vi "Show Front Panel.vi"(4 "Window Vertical Size (pixels)":i16=600, 6 "Window Horizontal Size (pixels)":i16=800, 8 "Error In":errorcluster, 10 "Window Behaviour":T1, 11 "VI Reference":refnum<vi>) -> (0 "Error Out":errorcluster)   [LabVIEW 2016, in "Error Manager.lvlib"]
doc: "This VI configures the front panel window of the Error Manager Main VI. This VI is expected to be called when the user presses the button that enables them to view the list of errors that may have occurred in the application up to that point."
uses:
  Error Manager.lvlib
  <vilib>/Utility/miscctls.llb/LVPointTypeDef.ctl
  <vilib>/Utility/miscctls.llb/LVRectTypeDef.ctl
  Settings/Window_Behaviour (enum).ctl
  Settings/Settings.lvclass
panel:
  # "Development\ncontrols/indicators useful for development and testing, but which are not outputs of the VI"
  # "Input\nInputs to the VI"
  # "Output\nOutputs of the VI"
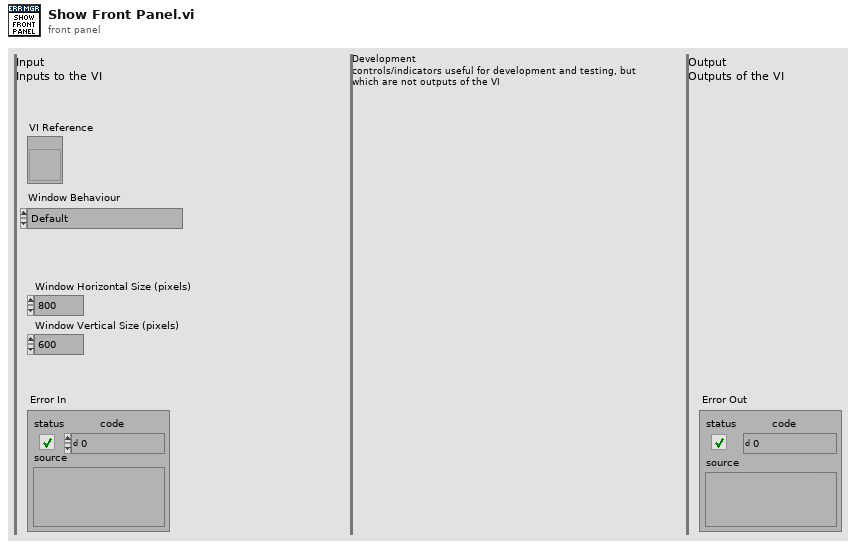
[diagram p1: front panel]
types:
  T1 = typedef "Error Manager.lvlib/Settings.lvclass/Window_Behaviour (enum).ctl" = enum16{"Default", "Floating", "Modal"}
  T2 = enum32{"Invalid", "Standard", "Closed", "Hidden", "Minimized", "Maximized"}
  T3 = typedef "LVRectTypeDef.ctl" = cluster{"Left":i16, "Top":i16, "Right":i16, "Bottom":i16}
  T4 = typedef "LVPointTypeDef.ctl" = cluster{"Horizontal":i16, "Vertical":i16}
  T5 = enum16{"Always On", "Always Off", "Off While Running"}
  T6 = enum32{"Invalid", "Default", "Floating", "Floating/Auto-Hide", "Modal"}
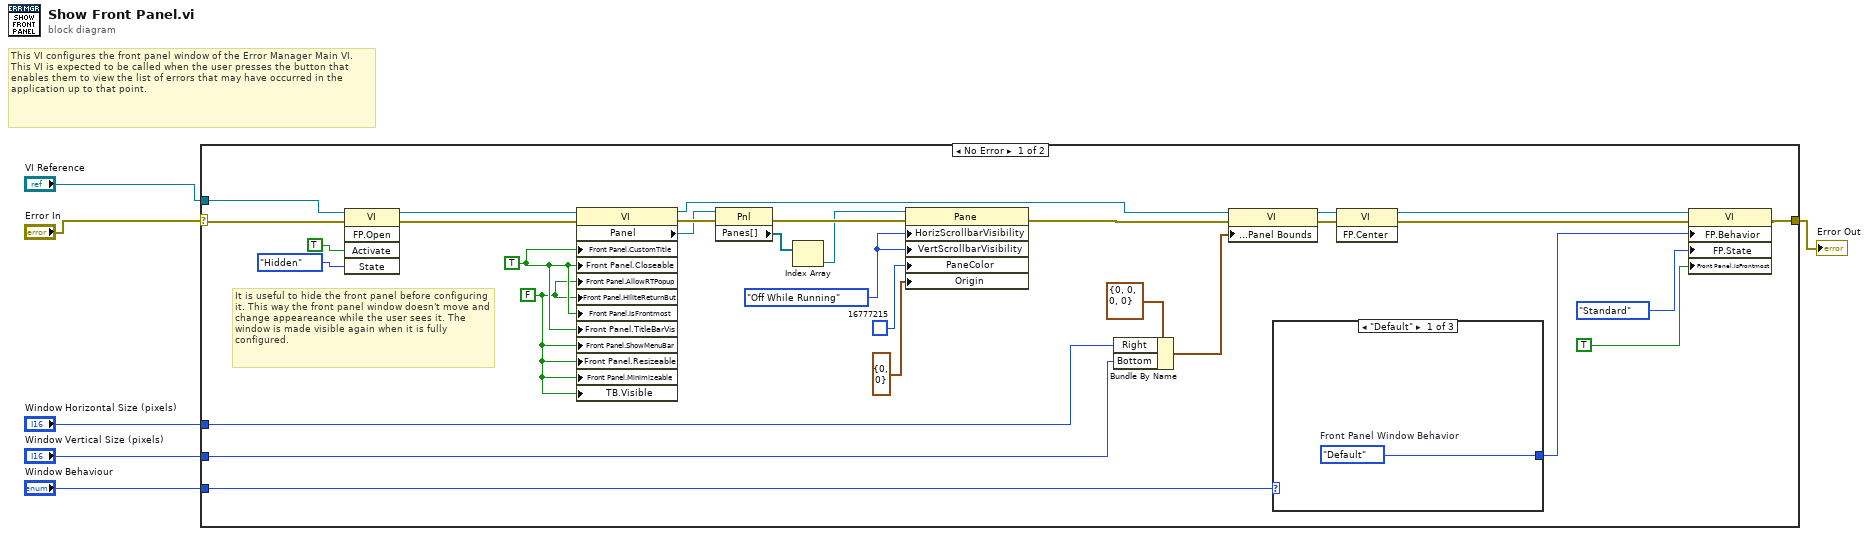
[diagram p0: block diagram]
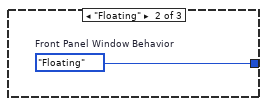
[diagram p2: hidden frame]
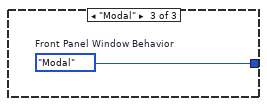
[diagram p3: hidden frame]
diagram:
  # "This VI configures the front panel window of the Error Manager Main VI. This VI is expected to be called when the user presses the button that enables them to view the list of errors that may have occurred in the application up to that point."
  n1 = case shown="No Error" "Error In" {
    selector: "Error In" -> [w17 w41]
    tunnel: [w10 w41] -> w4
    tunnel: "VI Reference" -> [w15 _]
    tunnel: "Window Horizontal Size (pixels)" -> [w21 _]
    tunnel: "Window Vertical Size (pixels)" -> [w20 _]
    tunnel: "Window Behaviour" -> [w8 _]
    frame No Error {
      w31 = T5."Off While Running" ("Horizontal Scrollbar Visibility")
      w29 = FALSE
      w36 = TRUE
      # "It is useful to hide the front panel before configuring it. This way the front panel window doesn't move and change appeareance while the user sees it. The window is made visible again when it is fully configured."
      n2 = invoke class="VI" method="FP.Open"(reference=w15, error in=w17, "Activate"=TRUE ("Activate?"), "State"=T2."Hidden") -> (reference out=w14:refnum<vi>, error out=w16:errorcluster)  [unwired: 1 in, 3 out]
      n3 = property class="VI"(reference=w14, error in=w16, "Front Panel.CustomTitle"=w36, "Front Panel.Closeable"=w36, "Front Panel.AllowRTPopup"=w29, "Front Panel.HiliteReturnBut"=w29, "Front Panel.IsFrontmost"=w36, "Front Panel.TitleBarVis"=w36, "Front Panel.ShowMenuBar"=w29, "Front Panel.Resizeable"=w29, "Front Panel.Minimizeable"=w29, "TB.Visible"=w29) -> (reference out=w25:refnum<vi>, error out=w37:errorcluster, "Panel"=w34:refnum<vi>)
      n4 = property class="Pnl"(reference=w34, error in=w37) -> (error out=w35:errorcluster, "Panes[]"=w33:refnum<vi>[])  [unwired: 1 out]
      n5 = Index Array(array=w33) -> (element=w32:refnum<vi>)  [unwired: 1 in]
      n6 = property class="Pane"(reference=w32, error in=w35, "HorizScrollbarVisibility"=w31, "VertScrollbarVisibility"=w31, "PaneColor"=u32 16777215, "Origin"=T4 {"Horizontal"=0, "Vertical"=0}) -> (error out=w27:errorcluster)  [unwired: 1 out]
      n7 = Bundle By Name(cluster=T3 {"Left"=0, "Top"=0, "Right"=0, "Bottom"=0} ("Front Panel Window:Panel Bounds"), "Right"=w21, "Bottom"=w20) -> (w23:T3)
      n8 = property on="Property Node" class="VI"(reference=w25, error in=w27, "Front Panel Window:Panel Bounds"=w23) -> (reference out=w22:refnum<vi>, error out=w26:errorcluster)
      n9 = case shown="\"Default\"" w8 {
        tunnel: [w38 w39 w40] -> w7
        frame "Default" {
          w38 = T6."Default"  # Front Panel Window Behavior
        }
        frame "Floating" {
          w39 = T6."Floating"  # Front Panel Window Behavior
        }
        frame "Modal" {
          w40 = T6."Modal"  # Front Panel Window Behavior
        }
      }
      n10 = invoke class="VI" method="FP.Center"(reference=w22, error in=w26) -> (reference out=w9:refnum<vi>, error out=w11:errorcluster)  [unwired: 1 in, 1 out]
      n11 = property class="VI"(reference=w9, error in=w11, "FP.Behavior"=w7, "FP.State"=T2."Standard" ("Front Panel Window:State"), "Front Panel.IsFrontmost"=TRUE ("Front Panel Window:Is Frontmost")) -> (error out=w10:errorcluster)  [unwired: 1 out]
    }
    frame Error {
    }
  }
  "Error Out" <- w4
